vi "Load Axis.vi"(8 "err in":errorcluster caption="エラー入力（エラーなし）", 11 "WaveformGraph入力":refnum<vi>) -> (0 "err out":errorcluster caption="エラー出力")   [LabVIEW 2014]
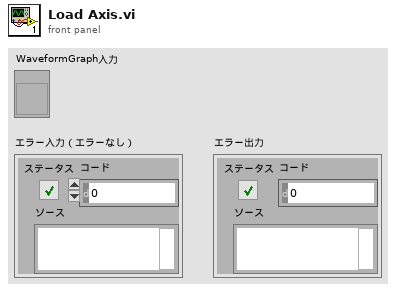
[diagram p1: front panel]
types:
  T1 = typedef "LVRangeTypeDef.ctl" = cluster{"Minimum":dbl, "Maximum":dbl, "Increment":dbl, "Minor Increment":dbl, "Start":dbl}
  T2 = cluster{"NameLbl.Text":string, "UnitLabel.Text":string, "Range":T1}
  T3 = cluster{cluster{"NameLbl.Text":string, "UnitLabel.Text":string, "Range":T1}[], cluster{"NameLbl.Text":string, "UnitLabel.Text":string, "Range":T1}[]}
  T4 = cluster{"NameLbl.Text":string, "UnitLabel.Text":string, "Range":T1}[]
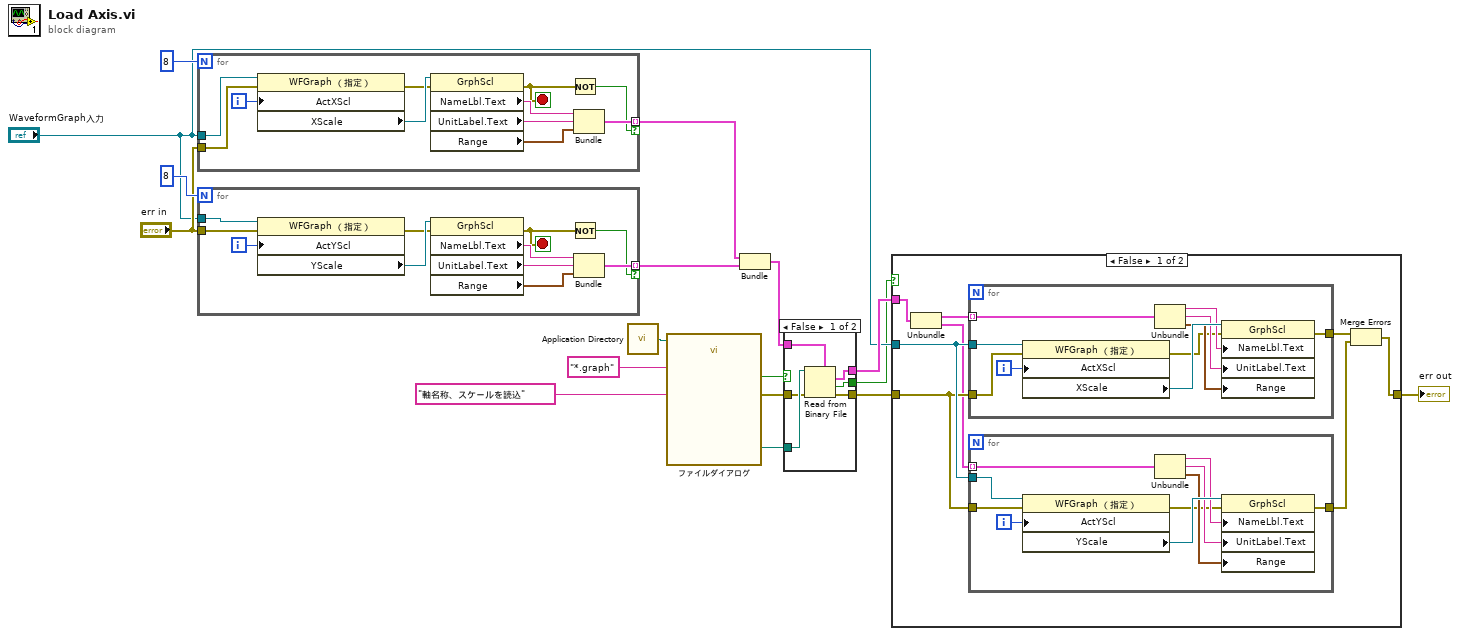
[diagram p0: block diagram]
diagram:
  n1 = for {
    N: 8 -> [_]
    tunnel: "err in" -> [w28]
    tunnel: "WaveformGraph入力" -> [w26]
    tunnel: [w22] -> w6 mode=indexing if=w18
    i -> [w21]
    stop <- w19 stop-if-true
    n2 = property class="WFGraph （指定）"(reference=w26, error in=w28, "ActXScl"=w21) -> (error out=w20:errorcluster, "XScale"=w27:refnum<vi>)  [unwired: 1 out]
    n3 = property class="GrphScl"(reference=w27, error in=w20) -> (error out=w19:errorcluster, "NameLbl.Text"=w25:string, "UnitLabel.Text"=w24:string, "Range"=w23:T1)  [unwired: 1 out]
    n4 = Not(x=w19) -> (.not. x?=w18:bool)
    n5 = Bundle("NameLbl.Text"=w25, "UnitLabel.Text"=w24, "Range"=w23) -> (w22:T2)  [unwired: 1 in]
  }
  n6 = for {
    N: 8 -> [_]
    tunnel: "err in" -> [w39]
    tunnel: "WaveformGraph入力" -> [w37]
    tunnel: [w33] -> w5 mode=indexing if=w29
    i -> [w32]
    stop <- w30 stop-if-true
    n7 = property class="WFGraph （指定）"(reference=w37, error in=w39, "ActYScl"=w32) -> (error out=w31:errorcluster, "YScale"=w38:refnum<vi>)  [unwired: 1 out]
    n8 = property class="GrphScl"(reference=w38, error in=w31) -> (error out=w30:errorcluster, "NameLbl.Text"=w36:string, "UnitLabel.Text"=w35:string, "Range"=w34:T1)  [unwired: 1 out]
    n9 = Not(x=w30) -> (.not. x?=w29:bool)
    n10 = Bundle("NameLbl.Text"=w36, "UnitLabel.Text"=w35, "Range"=w34) -> (w33:T2)  [unwired: 1 in]
  }
  n11 = call <vilib>:"Application Directory.vi"() -> ("Application Directory"=w14:path)
  n12 = call "ファイルダイアログ"("start path"=w14, "prompt"="軸名称、スケールを読込", "pattern (all files)"="*.graph") -> ("selected path"=w8:path, "cancelled"=w10:bool, "error out"=w9:errorcluster)  [unwired: 9 in, 1 out]
  n13 = Bundle(w6, w5) -> (w15:T3)  [unwired: 1 in]
  n14 = case shown="FALSE" w10 {
    selector: w10 -> [_ w46]
    tunnel: [w43 w47] -> w3
    tunnel: w15 -> [w42 _]
    tunnel: w9 -> [w44 w47]
    tunnel: w8 -> [w45 _]
    tunnel: [w41 _] -> w7
    tunnel: [w40 w46] -> w1
    frame False {
      n15 = Read from Binary File(5:w42, 8:w44, 11:w45) -> (0:w43:errorcluster, 1:w40:bool, 2:w41:T3)  [unwired: 3 in, 1 out]
    }
    frame True {
    }
  }
  n16 = case shown="FALSE" w1 {
    tunnel: w7 -> [w55 _]
    tunnel: "WaveformGraph入力" -> [w54 _]
    tunnel: w3 -> [w53 w76]
    tunnel: [w50 w76] -> w2
    frame False {
      n17 = Unbundle(w55) -> (w49:T4, w48:T4)
      n18 = for {
        tunnel: w49 -> [w72] mode=indexing
        tunnel: w54 -> [w74]
        tunnel: w53 -> [w68]
        tunnel: [w66] -> w52
        i -> [w75]
        n19 = property class="WFGraph （指定）"(reference=w74, error in=w68, "ActXScl"=w75) -> (error out=w67:errorcluster, "XScale"=w73:refnum<vi>)  [unwired: 1 out]
        n20 = Unbundle(w72) -> ("NameLbl.Text"=w71:string, "UnitLabel.Text"=w70:string, "Range"=w69:T1)
        n21 = property class="GrphScl"(reference=w73, error in=w67, "NameLbl.Text"=w71, "UnitLabel.Text"=w70, "Range"=w69) -> (error out=w66:errorcluster)  [unwired: 1 out]
      }
      n22 = for {
        tunnel: w48 -> [w62] mode=indexing
        tunnel: w54 -> [w64]
        tunnel: w53 -> [w58]
        tunnel: [w56] -> w51
        i -> [w65]
        n23 = property class="WFGraph （指定）"(reference=w64, error in=w58, "ActYScl"=w65) -> (error out=w57:errorcluster, "YScale"=w63:refnum<vi>)  [unwired: 1 out]
        n24 = Unbundle(w62) -> ("NameLbl.Text"=w61:string, "UnitLabel.Text"=w60:string, "Range"=w59:T1)
        n25 = property class="GrphScl"(reference=w63, error in=w57, "NameLbl.Text"=w61, "UnitLabel.Text"=w60, "Range"=w59) -> (error out=w56:errorcluster)  [unwired: 1 out]
      }
      n26 = Merge Errors(w52, w51) -> (w50:errorcluster)
    }
    frame True {
    }
  }
  "err out" <- w2
